vi "checkEXIT.vi"(11 "Path":string) -> (3 "EXIT?":bool)   [LabVIEW 2019]
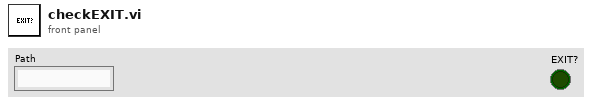
[diagram p1: front panel]
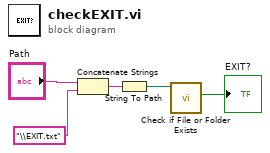
[diagram p0: block diagram]
diagram:
  n1 = Concatenate Strings("Path", "\\EXIT.txt" ("string")) -> (w4:string)
  n2 = String To Path(string=w4) -> (path=w3:path)
  n3 = call <vilib>:"Check if File or Folder Exists.vi"("path"=w3) -> ("file or folder exists?"=→"EXIT?":bool)  [unwired: 8 in, 2 out]
